vi "PololuGetCommand.vi"(4 "PololuCommand":T3="ReadModeStatus") -> (0 "Error":bool, 1 "CommandDescriptor":T1={"PololuCommand"="ReadModeStatus", "Mnemonic"="", "CommandType"=enum."Command", "Min"=0, "Max"=0})   [LabVIEW 2018]
uses:
  PololuCommandDescriptor.ctl
  TicCommandType.ctl
  PololuCommand.ctl
panel:
  in  "CommandDescriptorArray":T1[](array[typedef])=[{"PololuCommand"="SetTargetPosition", "Mnemonic"="à", "CommandType"=enum."32-bitWrite", "Min"=-2147483648, "Max"=2147483647}, {"PololuCommand"="SetTargetVelocity", "Mnemonic"="ã", "CommandType"=enum."32-bitWrite", "Min"=-500000000, "Max"=500000000}, {"PololuCommand"="HaltSetPosition", "Mnemonic"="ì", "CommandType"=enum."32-bitWrite", "Min"=-2147483648, "Max"=2147483647}, {"PololuCommand"="HaltHold", "Mnemonic"="‰", "CommandType"=enum."Command", "Min"=0, "Max"=0}, {"PololuCommand"="ResetTimeout", "Mnemonic"="Œ", "CommandType"=enum."Command", "Min"=0, "Max"=0}, {"PololuCommand"="De-energize", "Mnemonic"="†", "CommandType"=enum."Command", "Min"=0, "Max"=0}, {"PololuCommand"="Energize", "Mnemonic"="…", "CommandType"=enum."Command", "Min"=0, "Max"=0}, {"PololuCommand"="ExitSafeStart", "Mnemonic"="ƒ", "CommandType"=enum."Command", "Min"=0, "Max"=0}, {"PololuCommand"="EnterSafeStart", "Mnemonic"="", "CommandType"=enum."Command", "Min"=0, "Max"=0}, {"PololuCommand"="Reset", "Mnemonic"="°", "CommandType"=enum."Command", "Min"=0, "Max"=0}, {"PololuCommand"="ClearDriverError", "Mnemonic"="Š", "CommandType"=enum."Command", "Min"=0, "Max"=0}, {"PololuCommand"="SetMaxSpeed", "Mnemonic"="æ", "CommandType"=enum."32-bitWrite", "Min"=0, "Max"=500000000}, {"PololuCommand"="SetStartSpeed", "Mnemonic"="å", "CommandType"=enum."32-bitWrite", "Min"=0, "Max"=500000000}, {"PololuCommand"="SetMaxAcc", "Mnemonic"="ê", "CommandType"=enum."32-bitWrite", "Min"=100, "Max"=2147483647}, {"PololuCommand"="SetMaxDec", "Mnemonic"="é", "CommandType"=enum."32-bitWrite", "Min"=0, "Max"=2147483647}, {"PololuCommand"="SetStepMode", "Mnemonic"="”", "CommandType"=enum."7-bitWrite", "Min"=0, "Max"=5}, {"PololuCommand"="SetCurrLim", "Mnemonic"="‘", "CommandType"=enum."7-bitWrite", "Min"=0, "Max"=124}, {"PololuCommand"="SetDecayMode", "Mnemonic"="’", "CommandType"=enum."7-bitWrite", "Min"=0, "Max"=4}, {"PololuCommand"="GetVar", "Mnemonic"="¡", "CommandType"=enum."BlockRead", "Min"=0, "Max"=81}, {"PololuCommand"="GetVarClrErr", "Mnemonic"="¢", "CommandType"=enum."BlockRead", "Min"=0, "Max"=81}, {"PololuCommand"="GetSetting", "Mnemonic"="¨", "CommandType"=enum."BlockRead", "Min"=0, "Max"=94}, {"PololuCommand"="ReadModeStatus", "Mnemonic"="", "CommandType"=enum."Command", "Min"=0, "Max"=0}]
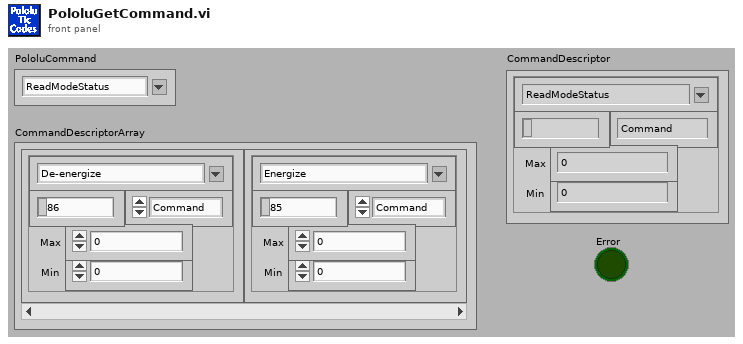
[diagram p1: front panel]
types:
  T1 = typedef "PololuCommandDescriptor.ctl" = cluster{"PololuCommand":string, "Mnemonic":string, "CommandType":T2, "Min":i32, "Max":i32}
  T2 = typedef "TicCommandType.ctl" = enum16{"Command", "7-bitWrite", "32-bitWrite", "BlockRead"}
  T3 = typedef "PololuCommand.ctl" = string
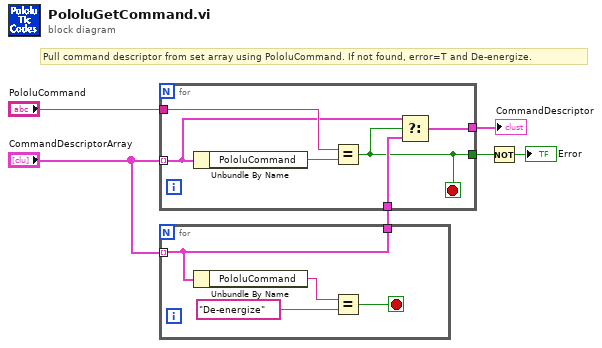
[diagram p0: block diagram]
diagram:
  # "Pull command descriptor from set array using PololuCommand. If not found, error=T and De-energize."
  n1 = for {
    tunnel: "CommandDescriptorArray" -> [w8] mode=indexing
    tunnel: [w8] -> w2
    stop <- w9 stop-if-true
    n2 = Unbundle By Name(w8) -> ("PololuCommand"=w10:string)
    n3 = Equal?(x=w10, y="De-energize" ("PololuCommand")) -> (x = y?=w9:bool)
  }
  n4 = for {
    tunnel: "CommandDescriptorArray" -> [w13] mode=indexing
    tunnel: "PololuCommand" -> [w15]
    tunnel: [w14] -> w1
    tunnel: w2 -> [w12]
    tunnel: [w11] -> w6
    stop <- w11 stop-if-true
    n5 = Unbundle By Name(w13) -> ("PololuCommand"=w16:string)
    n6 = Equal?(x=w15, y=w16) -> (x = y?=w11:bool)
    n7 = Select(t=w13, s=w11, f=w12) -> (s? t:f=w14:T1)
  }
  "CommandDescriptor" <- w1
  n8 = Not(x=w6) -> (.not. x?=→"Error":bool)
